vi "Initialize.vi"(8 "error in (no error)":errorcluster, 11 "Ismatech 3 Channel Settings In":T1 {"Channel Number" min=0 max=3; "Pump Number" min=1 max=9}) -> (0 "error out":errorcluster, 1 "Initialized":bool, 2 "No Pump Connected":bool=TRUE, 3 "Ismatech 3 Channel Settings Out":T1={"VISA resource name"="", "Pump Number"=1, "Channel Number"=0, "Simulated?"=TRUE, "Reverse?"=FALSE} {"Channel Number" min=0 max=3; "Pump Number" min=1 max=9})   [LabVIEW 2018, in "Ismatec 4308.lvlib"]
uses:
  Ismatec 4308.lvlib
  Ismatec 4083.ctl
  <vilib>/Instr/_visa.llb/VISA Configure Serial Port (Instr).vi
  support/Support Library.lvlib
panel:
  out "read 4":string
  out "read buffer 3":string
  out "read buffer 2":string
  out "read buffer":string
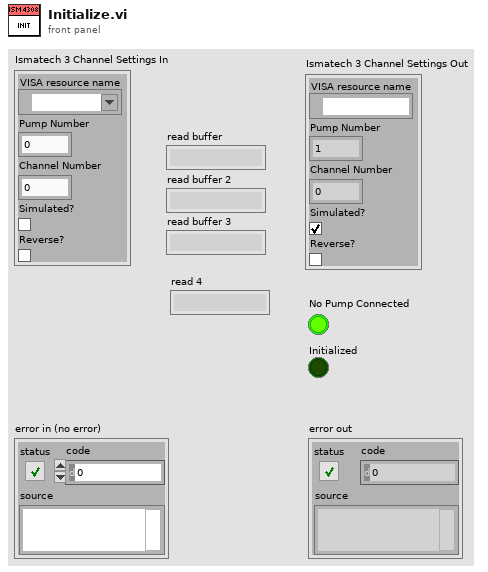
[diagram p1: front panel]
types:
  T1 = typedef "Ismatec 4308.lvlib/Ismatec 4083.ctl" = cluster{"VISA resource name":refnum<visa-resource-name>, "Pump Number":i16, "Channel Number":i16, "Simulated?":bool, "Reverse?":bool}
  T2 = typedef "Ismatec 4308.lvlib/Ismatec 4083 Global.ctl" = T3[]
  T3 = typedef "Ismatec 4308.lvlib/Ismatec 4083 Global Element.ctl" = cluster{"Busy":bool, "ChannelCnt":dbl, "Initialized":bool, "Current Channel":dbl, "Initialized Channels":dbl[]}
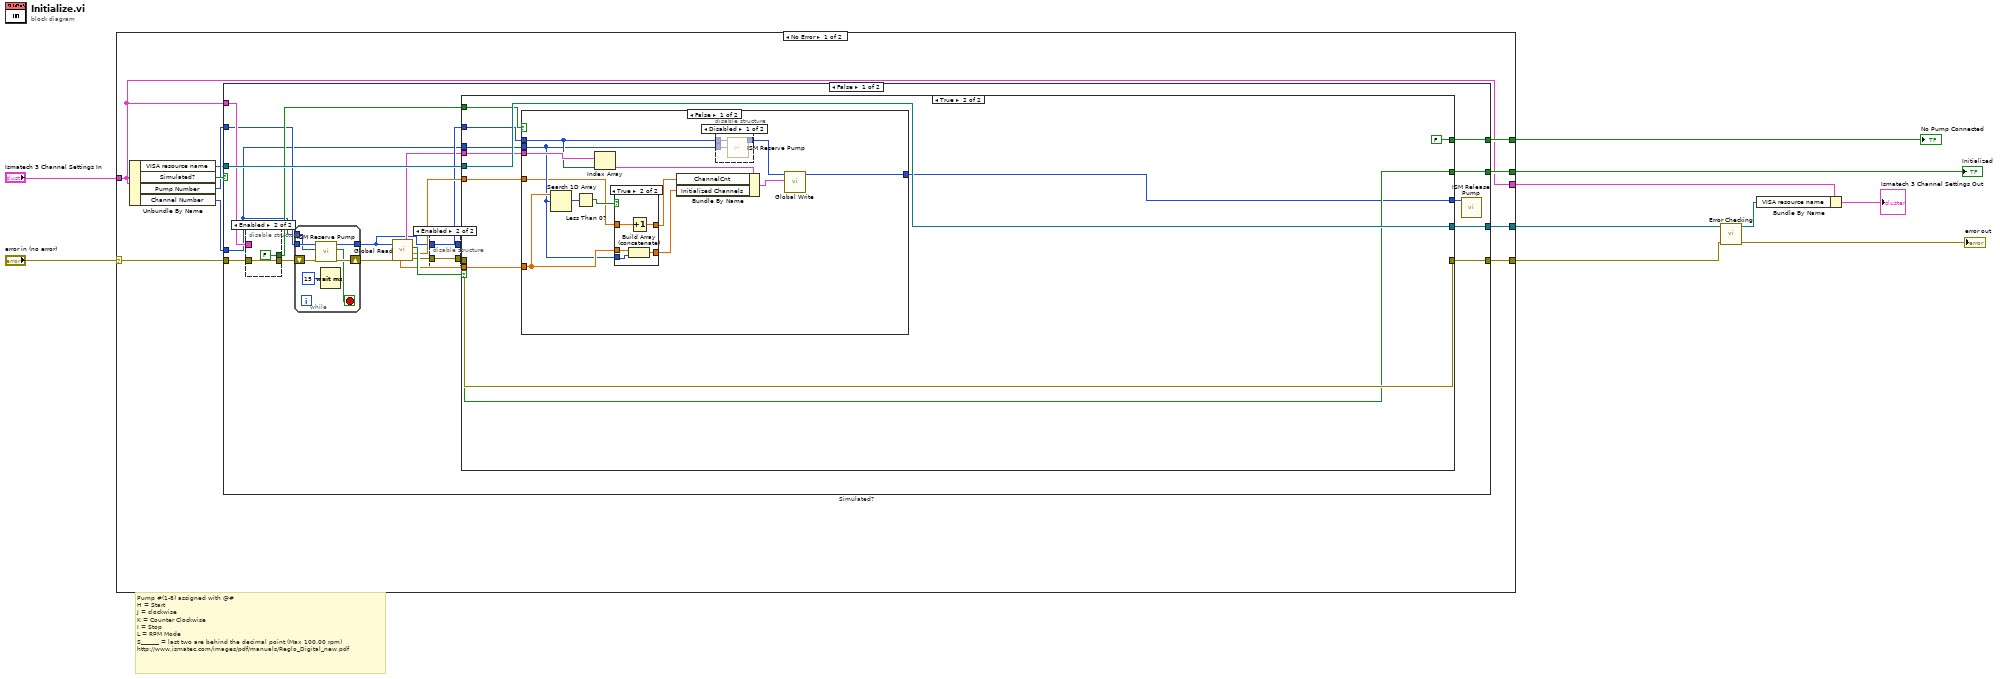
[diagram p0: block diagram]
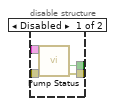
[diagram p2: hidden frame]
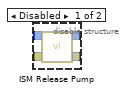
[diagram p3: hidden frame]
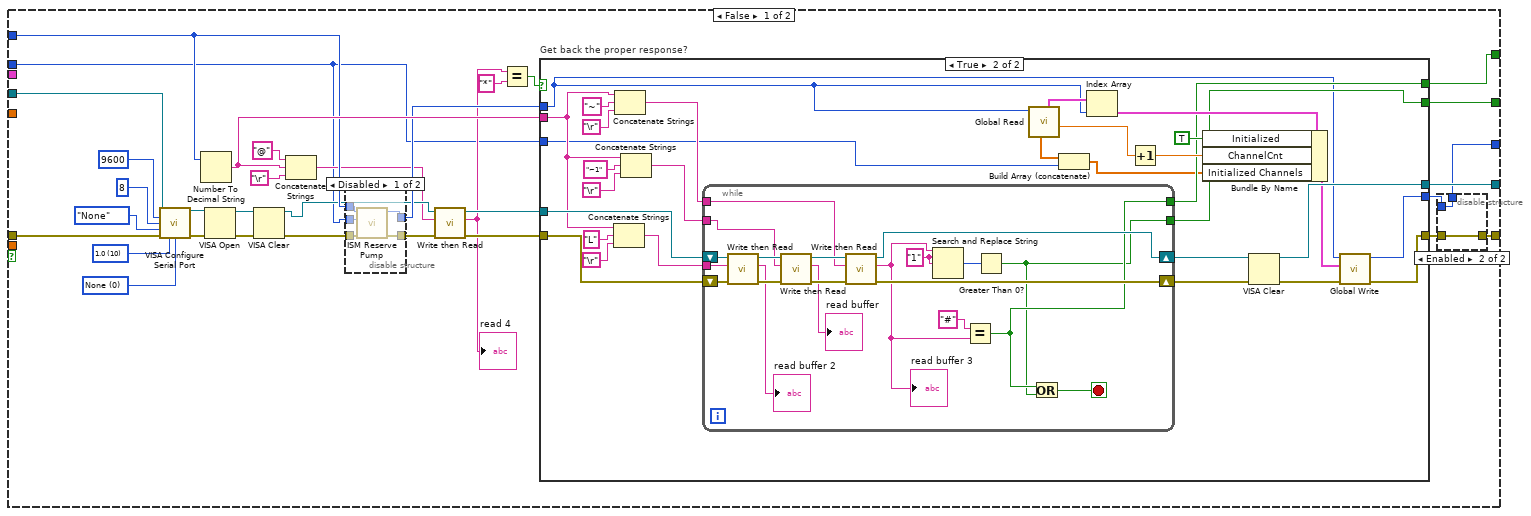
[diagram p4: hidden frame]
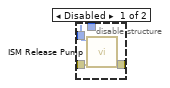
[diagram p6: hidden frame]
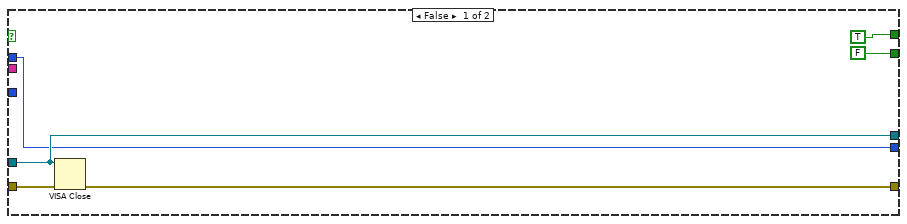
[diagram p7: hidden frame]
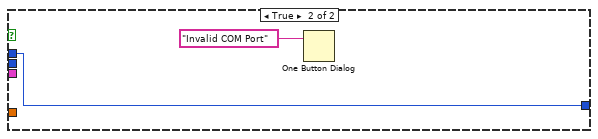
[diagram p10: hidden frame]
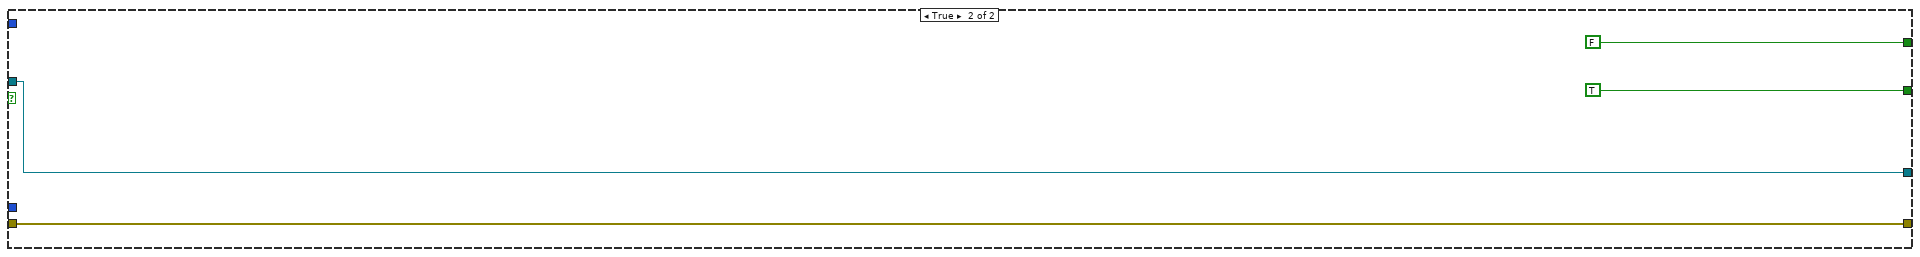
[diagram p11: hidden frame]
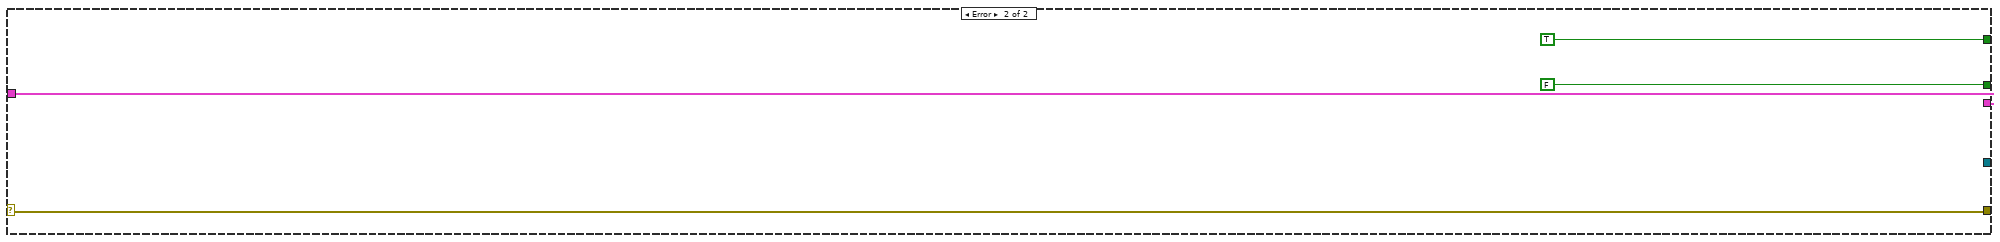
[diagram p12: hidden frame]
diagram:
  # "Pump #(1-8) assigned with @#\nH = Start\nJ = clockwise\nK = Counter Clockwise\nI = Stop\nL = RPM Mode\nS______ = last two are behind the decimal point (Max 100.00 rpm)\nhttp://www.ismatec.com/images/pdf/manuals/Reglo_Digital_new.pdf"
  n1 = case shown="No Error" "error in (no error)" {
    selector: "error in (no error)" -> [w16 w206]
    tunnel: "Ismatech 3 Channel Settings In" -> [w12 w205]
    tunnel: [w19 w206] -> w7
    tunnel: [w12 w205] -> w6
    tunnel: [w15 _] -> w5
    tunnel: [w14 FALSE] -> w4
    tunnel: [w13 TRUE] -> w1
    frame No Error {
      n2 = Unbundle By Name(w12) -> ("VISA resource name"=w17:refnum<visa-resource-name>, "Simulated?"=w20:bool, "Pump Number"=w18:i16, "Channel Number"=w11:i16)
      n3 = case "Simulated?" shown="False" w20 {
        tunnel: [w38 w201] -> w19
        tunnel: [w39 w202] -> w15
        tunnel: w18 -> [w25 _]
        tunnel: w17 -> [w41 w202]
        tunnel: w16 -> [w27 w201]
        tunnel: [w40 TRUE] -> w14
        tunnel: [w35 FALSE] -> w13
        tunnel: w12 -> [w29 _]
        tunnel: w11 -> [w24 _]
        frame False {
          n4 = disable-structure shown="Enabled" {
            disable-tunnel: w29 -> [w52 _]
            disable-tunnel: [w51 FALSE ("Connection Error")] -> w28
            disable-tunnel: w27 -> [w50 w54]
            disable-tunnel: [w49 w54] -> w21
            frame Disabled {
              n5 = call "Pump Status.vi"("error in (no error)"=w50, "Ismatech 3 Channel Settings In"=w52) -> ("error out"=w49:errorcluster, "Connection Error"=w51:bool)  [unwired: 5 in, 3 out]
            }
            frame Enabled {
            }
          }
          n6 = while {
            tunnel: w25 -> [w46]
            tunnel: w24 -> [w45]
            shift-right: [w47] -> w22
            shift-left: w21 -> [w48]
            tunnel: [w42] -> w23
            stop <- w44 stop-if-true
            n7 = call "ISM Reserve Pump.vi"("error in (no error)"=w48, "ISM Channel # In"=w45, "ISM Pump # In"=w46) -> ("error out"=w47:errorcluster, "Loop Completed"=w44:bool, "ISM Pump # Out"=w42:i32)  [unwired: 6 in]
            n8 = Wait (ms)(milliseconds to wait=u32 15) -> ()  [unwired: 1 out]
          }
          n9 = call "Global Read.vi"("error in (no error)"=w22, "Pump Number"=w23) -> ("error out"=w34:errorcluster, "ChannelCnt"=w36:dbl, "Initialized"=w37:bool, "Ismatec 4083 Global"=w31:T2, "Initialized Channels"=w30:dbl[])  [unwired: 3 in, 2 out]
          n10 = disable-structure shown="Enabled" {
            disable-tunnel: w23 -> [w58 w60]
            disable-tunnel: w34 -> [w57 w59]
            disable-tunnel: [w56 w59] -> w33
            disable-tunnel: [w55 w60] -> w32
            frame Disabled {
              n11 = call "ISM Release Pump.vi"("error in (no error)"=w57, "Pump Number In"=w58) -> ("error out"=w56:errorcluster, "Pump Number Out"=w55:i32)  [unwired: 8 in]
            }
            frame Enabled {
            }
          }
          n12 = case shown="True" w37 {
            selector: w37 -> [_ w170]
            tunnel: w41 -> [w89 w172]
            tunnel: w33 -> [w88 w171]
            tunnel: [w87 w170] -> w40
            tunnel: [w86 w172] -> w39
            tunnel: [w85 w171] -> w38
            tunnel: w32 -> [w84 w166]
            tunnel: w31 -> [_ w169]
            tunnel: w36 -> [_ w168]
            tunnel: [w83 FALSE] -> w35
            tunnel: w24 -> [w62 w165]
            tunnel: w30 -> [_ w164]
            tunnel: w28 -> [_ w163]
            tunnel: [w61 w162] -> w26
            frame False {
              w73 = u16 0 items=["None", "XON/XOFF", "RTS/CTS", "XON/XOFF & RTS/CTS", "DTR/DSR", "XON/XOFF & DTR/DSR"] ("flow control (0:none)")
              w74 = u16 10 items=["1.0"=10, "1.5"=15, "2.0"=20] ("stop bits (10: 1 bit)")
              n13 = call-poly "VISA Configure Serial Port"("VISA resource name"=w89, "baud rate (9600)"=u32 9600, "data bits (8)"=u16 8, "parity (0:none)"=enum16{"None", "Odd", "Even", "Mark", "Space"}."None", "error in (no error)"=w88, "stop bits (10: 1 bit)"=w74, "flow control (0:none)"=w73) -> ("VISA resource name out"=w81:refnum<visa-resource-name>, "error out"=w80:errorcluster)  [unwired: 7 in]
              n14 = Number To Decimal String(number=w84) -> (decimal integer string=w91:string)  [unwired: 1 in]
              n15 = VISA Open(error in (no error)=w80, VISA resource name=w81) -> (VISA resource name=w72:refnum<visa-resource-name>, error out=w71:errorcluster)  [unwired: 3 in]
              n16 = VISA Clear(VISA resource name=w72, error in (no error)=w71) -> (VISA resource name out=w69:refnum<visa-resource-name>, error out=w70:errorcluster)
              n17 = Concatenate Strings("@" ("string"), w91, "\r") -> (w68:string)
              n18 = disable-structure shown="Disabled" {
                disable-tunnel: [w98 w100] -> w90
                disable-tunnel: w84 -> [w97 w100]
                disable-tunnel: w70 -> [w96 w99]
                disable-tunnel: [w95 w99] -> w67
                disable-tunnel: w62 -> [w94 _]
                frame Disabled {
                  n19 = call "ISM Reserve Pump.vi"("error in (no error)"=w96, "ISM Channel # In"=w94, "ISM Pump # In"=w97) -> ("error out"=w95:errorcluster, "ISM Pump # Out"=w98:i32)  [unwired: 6 in, 1 out]
                }
                frame Enabled {
                }
              }
              n20 = call "Write then Read.vi"("error in"=w67, "write buffer"=w68, "VISA resource name in"=w69) -> ("error out"=w92:errorcluster, "read buffer"=w82:string, "VISA resource name out"=w93:refnum<visa-resource-name>)  [unwired: 6 in]
              "read 4" <- w82
              n21 = Equal?(x=w82, y="*") -> (x = y?=w65:bool)
              n22 = case "Get back the proper response?" shown="True" w65 {
                tunnel: w93 -> [w107 w141]
                tunnel: w92 -> [w111 w140]
                tunnel: [w110 w124] -> w63
                tunnel: [TRUE w118] -> w83
                tunnel: [FALSE w119] -> w87
                tunnel: [w107 w135] -> w86
                tunnel: w91 -> [_ w117]
                tunnel: [w106 w126] -> w64
                tunnel: w90 -> [w106 w115]
                tunnel: w62 -> [_ w112]
                frame False {
                  n23 = VISA Close(VISA resource name=w107, error in (no error)=w111) -> (error out=w110:errorcluster)
                }
                frame True {
                  n24 = Concatenate Strings(w117, "L" ("string"), "\r") -> (w137:string)
                  n25 = Concatenate Strings(w117, "~" ("string"), "\r") -> (w120:string)
                  n26 = Concatenate Strings(w117, "~1" ("string"), "\r") -> (w134:string)
                  n27 = while {
                    tunnel: w137 -> [w151]
                    tunnel: w134 -> [w150]
                    shift-right: [w156] -> w132
                    shift-left: w141 -> [w159]
                    shift-right: [w155] -> w133
                    shift-left: w140 -> [w152]
                    tunnel: w120 -> [w149]
                    tunnel: [w145] -> w119
                    tunnel: [w146] -> w118
                    stop <- w160 stop-if-true
                    w143 = "1" ("search string")
                    n28 = call "Write then Read.vi"("error in"=w152, "write buffer"=w151, "VISA resource name in"=w159) -> ("error out"=w153:errorcluster, "read buffer"=→"read buffer 2":string, "VISA resource name out"=w158:refnum<visa-resource-name>)  [unwired: 6 in]
                    n29 = call "Write then Read.vi"("error in"=w153, "write buffer"=w150, "VISA resource name in"=w158) -> ("error out"=w154:errorcluster, "read buffer"=→"read buffer":string, "VISA resource name out"=w157:refnum<visa-resource-name>)  [unwired: 6 in]
                    n30 = call "Write then Read.vi"("error in"=w154, "write buffer"=w149, "VISA resource name in"=w157) -> ("error out"=w155:errorcluster, "read buffer"=w144:string, "VISA resource name out"=w156:refnum<visa-resource-name>)  [unwired: 6 in]
                    "read buffer 3" <- w144
                    n31 = Search and Replace String(input string=w144, search string=w143, replace string=w143) -> (number of replacements=w142:i32)  [unwired: 5 in, 3 out]
                    n32 = Equal?(x="#", y=w144) -> (x = y?=w146:bool)
                    n33 = Greater Than 0?(x=w142) -> (x > 0?=w145:bool)
                    n34 = Or(x=w146, y=w145) -> (x .or. y?=w160:bool)
                  }
                  n35 = call "Global Read.vi"("Pump Number"=w115) -> ("ChannelCnt"=w131:dbl, "Ismatec 4083 Global"=w116:T2, "Initialized Channels"=w114:dbl[])  [unwired: 4 in, 4 out]
                  n36 = Build Array (concatenate)(w114, w112) -> (w113:dbl[])
                  n37 = Index Array(array=w116, index=w115) -> (element=w130:T3)
                  n38 = Increment(x=w131) -> (x+1=w128:dbl)
                  n39 = Bundle By Name(cluster=w130, "Initialized"=TRUE, "ChannelCnt"=w128, "Initialized Channels"=w113) -> (w127:T3)
                  n40 = VISA Clear(VISA resource name=w132, error in (no error)=w133) -> (VISA resource name out=w135:refnum<visa-resource-name>, error out=w125:errorcluster)
                  n41 = call "Global Write.vi"("error in (no error)"=w125, "Incoming Cluster"=w127, "Pump Number In"=w115) -> ("error out"=w124:errorcluster, "Pump Number Out"=w126:i32)  [unwired: 7 in]
                }
              }
              n42 = disable-structure shown="Enabled" {
                disable-tunnel: [w103 w104] -> w85
                disable-tunnel: w64 -> [w102 w105]
                disable-tunnel: w63 -> [w101 w104]
                disable-tunnel: [_ w105] -> w61
                frame Disabled {
                  n43 = call "ISM Release Pump.vi"("error in (no error)"=w101, "Pump Number In"=w102) -> ("error out"=w103:errorcluster)  [unwired: 8 in, 1 out]
                }
                frame Enabled {
                }
              }
            }
            frame True {
              n44 = case shown="False" w163 {
                tunnel: w169 -> [w183 _]
                tunnel: w168 -> [w175 _]
                tunnel: w166 -> [w181 w197]
                tunnel: w165 -> [w178 _]
                tunnel: w164 -> [w179 _]
                tunnel: [w173 w197] -> w162
                frame False {
                  n45 = Search 1D Array(1D array=w179, element=w178) -> (index of element=w180:i32)  [unwired: 1 in]
                  n46 = Less Than 0?(x=w180) -> (x < 0?=w176:bool)
                  n47 = Index Array(array=w183, index=w181) -> (element=w184:T3)
                  n48 = case shown="True" w176 {
                    tunnel: w179 -> [w191 w196]
                    tunnel: w178 -> [_ w195]
                    tunnel: [w191 w194] -> w177
                    tunnel: w175 -> [w190 w193]
                    tunnel: [w190 w192] -> w174
                    frame False {
                    }
                    frame True {
                      n49 = Build Array (concatenate)(w196, w195) -> (w194:dbl[])
                      n50 = Increment(x=w193) -> (x+1=w192:dbl)
                    }
                  }
                  n51 = Bundle By Name(cluster=w184, "ChannelCnt"=w174, "Initialized Channels"=w177) -> (w185:T3)
                  n52 = disable-structure shown="Disabled" {
                    disable-tunnel: [w188 w189] -> w182
                    disable-tunnel: w181 -> [w187 w189]
                    disable-tunnel: w178 -> [w186 _]
                    frame Disabled {
                      n53 = call "ISM Reserve Pump.vi"("ISM Channel # In"=w186, "ISM Pump # In"=w187) -> ("ISM Pump # Out"=w188:i32)  [unwired: 7 in, 2 out]
                    }
                    frame Enabled {
                    }
                  }
                  n54 = call "Global Write.vi"("Incoming Cluster"=w185, "Pump Number In"=w182) -> ("Pump Number Out"=w173:i32)  [unwired: 8 in, 1 out]
                }
                frame True {
                  n55 = One Button Dialog(message="Invalid COM Port") -> ()  [unwired: 1 in, 1 out]
                }
              }
            }
          }
          n56 = call "ISM Release Pump.vi"("Pump Number In"=w26) -> ()  [unwired: 9 in, 2 out]
        }
        frame True {
        }
      }
    }
    frame Error {
    }
  }
  "Initialized" <- w4
  "No Pump Connected" <- w1
  n57 = call "Error Checking.vi"("error in (no error)"=w7, "VISA resource name"=w5) -> ("error out"=→"error out":errorcluster, "VISA resource name"=w9:refnum<visa-resource-name>)  [unwired: 7 in, 1 out]
  n58 = Bundle By Name(cluster=w6, "VISA resource name"=w9) -> (→"Ismatech 3 Channel Settings Out":T1)
